vi "Get State Diagram Reference.vi"(7 "Make Frame Visible?":bool, 8 "error in (no error)":errorcluster, 9 "State Name":string, 10 "Category (Optional)":string, 11 "JKI SM in":refnum<class "JKI SM.lvclass">) -> (0 "error out":errorcluster, 1 "index of Frame":i32, 2 "Frame Reference":refnum<vi>, 3 "JKI SM out":refnum<class "JKI SM.lvclass">, 5 "Found?":bool)   [LabVIEW 2020, in "JKI State Machine API.lvlib" / "JKI SM.lvclass"]
uses:
  JKI SM.lvclass
  JKI SM.lvclass/JKI SM.ctl
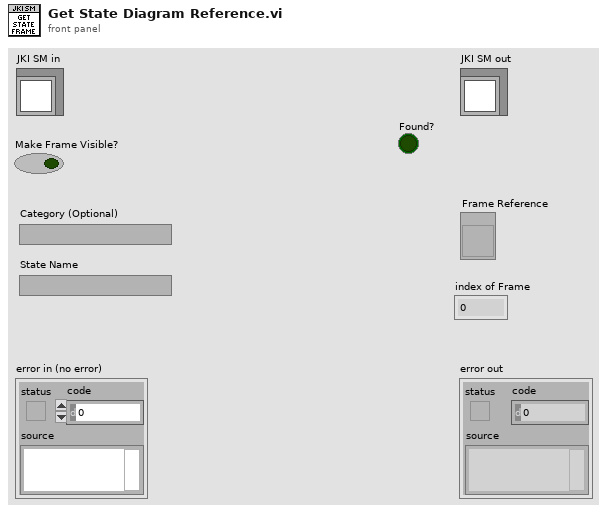
[diagram p1: front panel]
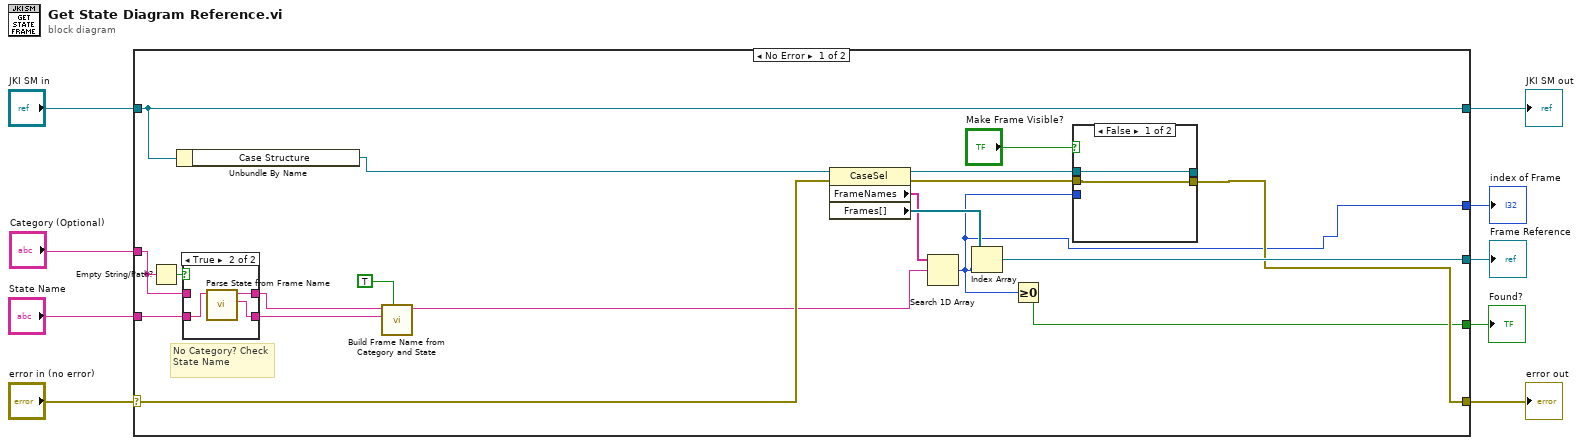
[diagram p0: block diagram]
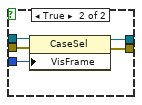
[diagram p2: hidden frame]
diagram:
  n1 = case shown="No Error" "error in (no error)" {
    selector: "error in (no error)" -> [w28 w42]
    tunnel: [w14 w42] -> w8
    tunnel: [w21 w41] -> w6
    tunnel: "JKI SM in" -> [w21 w41]
    tunnel: "State Name" -> [w24 _]
    tunnel: "Category (Optional)" -> [w25 _]
    tunnel: [w17 _] -> w3
    tunnel: [w11 _] -> w2
    tunnel: [w10 _] -> w1
    frame No Error {
      # "No Category? Check State Name"
      n2 = Empty String/Path?(string/path=w25) -> (empty?=w26:bool)
      n3 = Unbundle By Name(w21) -> ("Case Structure"=w27:refnum<vi>)
      n4 = case shown="True" w26 {
        tunnel: w24 -> [w36 w40]
        tunnel: [w37 w39] -> w22
        tunnel: w25 -> [w37 _]
        tunnel: [w36 w38] -> w23
        frame False {
        }
        frame True {
          n5 = call "Parse State from Frame Name.vi"("Frame or State Name"=w40) -> ("State Name"=w38:string, "Category Name"=w39:string)  [unwired: 5 in, 4 out]
        }
      }
      n6 = call "Build Frame Name from Category and State.vi"("Wrap in Quotes? (TRUE)"=TRUE, "State Name"=w23, "Category"=w22) -> ("Frame Name"=w20:string)  [unwired: 8 in]
      n7 = property class="CaseSel"(reference=w27, error in=w28) -> (reference out=w16:refnum<vi>, error out=w15:errorcluster, "FrameNames"=w18:string[], "Frames[]"=w19:refnum<vi>[])
      n8 = Search 1D Array(1D array=w18, element=w20) -> (index of element=w11:i32)  [unwired: 1 in]
      n9 = Index Array(array=w19, index=w11) -> (element=w17:refnum<vi>)
      n10 = Greater Or Equal To 0?(x=w11) -> (x >= 0?=w10:bool)
      n11 = case shown="False" "Make Frame Visible?" {
        tunnel: [w30 w35] -> _
        tunnel: [w29 w34] -> w14
        tunnel: w16 -> [w30 w33]
        tunnel: w15 -> [w29 w32]
        tunnel: w11 -> [_ w31]
        frame False {
        }
        frame True {
          n12 = property class="CaseSel"(reference=w33, error in=w32, "VisFrame"=w31) -> (reference out=w35:refnum<vi>, error out=w34:errorcluster)
        }
      }
    }
    frame Error {
    }
  }
  "error out" <- w8
  "JKI SM out" <- w6
  "Frame Reference" <- w3
  "index of Frame" <- w2
  "Found?" <- w1
